vi "ModifyGraph axThick.vi"(8 "error in (no error)":errorcluster, 10 "Axes Thickness (points) [0.5]":T1={"bottom"=0.5, "top"=0.5, "left"=0.5, "right"=0.5}, 11 "ITX Commands in":refnum<class "ITX Commands.lvclass">) -> (0 "error out":errorcluster, 3 "ITX Commands out":refnum<class "ITX Commands.lvclass">)   [LabVIEW 2016, in "ITX Commands.lvclass"]
uses:
  ITX Commands.lvclass
  ITX Commands.lvclass/ITX Commands.ctl
panel:
  out "resulting string":string
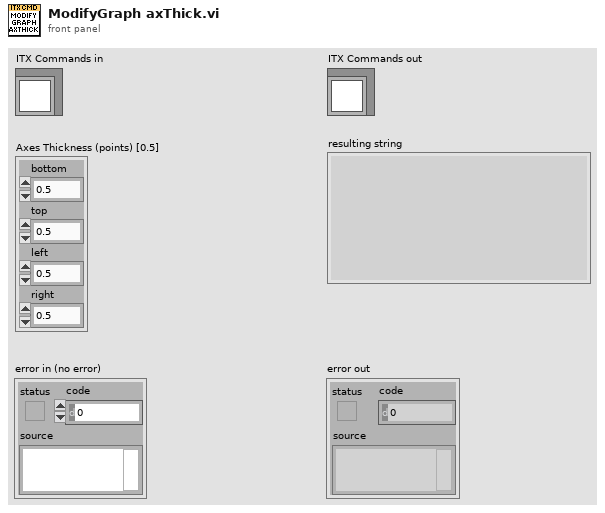
[diagram p1: front panel]
types:
  T1 = cluster{"bottom":dbl, "top":dbl, "left":dbl, "right":dbl}
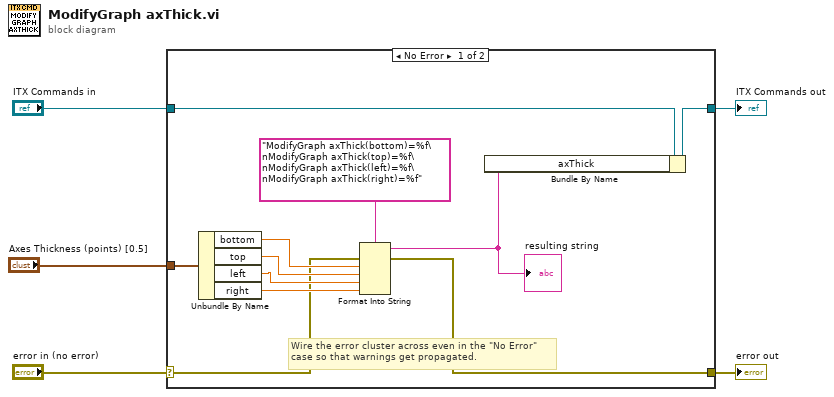
[diagram p0: block diagram]
diagram:
  n1 = case shown="No Error" "error in (no error)" {
    selector: "error in (no error)" -> [w7 w18]
    tunnel: [w6 w18] -> w4
    tunnel: [w8 w17] -> w2
    tunnel: "ITX Commands in" -> [w10 w17]
    tunnel: "Axes Thickness (points) [0.5]" -> [w16 _]
    frame No Error {
      # "Wire the error cluster across even in the \"No Error\"\ncase so that warnings get propagated."
      n2 = Unbundle By Name(w16) -> ("bottom"=w12:dbl, "top"=w13:dbl, "left"=w14:dbl, "right"=w15:dbl)
      n3 = Format Into String(format string="ModifyGraph axThick(bottom)=%f\nModifyGraph axThick(top)=%f\nModifyGraph axThick(left)=%f\nModifyGraph axThick(right)=%f", error in=w7, w12, w13, w14, w15) -> (resulting string=w9:string, error out=w6:errorcluster)  [unwired: 1 in]
      "resulting string" <- w9
      n4 = Bundle By Name(cluster=w10, "axThick"=w9) -> (w8:refnum<class "ITX Commands.lvclass">)
    }
    frame Error {
    }
  }
  "error out" <- w4
  "ITX Commands out" <- w2
